vi "Read Tester.vi"(6 "Maximum Time (10000 ms)":u32=10000, 8 "error in (no error)":errorcluster, 11 "VISA resource name":refnum<visa-resource-name>) -> (0 "error out":errorcluster, 1 "Current (A)":dbl format="%^#_9g", 2 "Power (dBm)":dbl format="%^#_9g", 3 "VISA resource name out":refnum<visa-resource-name>, 5 "Frequency (Hz)":dbl format="%^#_9g")   [LabVIEW 2011, in "Agilent E5052X.lvlib"]
doc: "Reads tester mode trace data of the Frequency/Power measurement from the instrument.\n\n<b>Note: </b>\n\nThis VI only applies to when the Frequency/Power mode has been set to \"Tester Mode\" instead of \"Analyzer Mode\" through the \"Configure Measurement (Freq-Power)\" VI."
uses:
  Agilent E5052X.lvlib
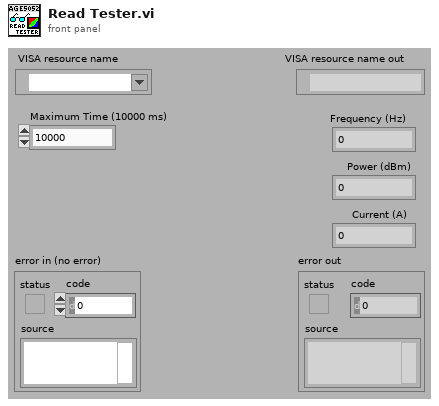
[diagram p1: front panel]
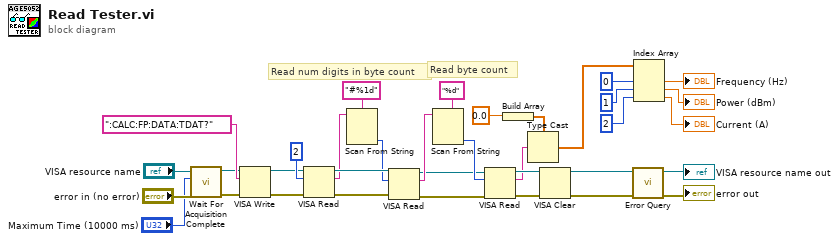
[diagram p0: block diagram]
diagram:
  # "Read num digits in byte count"
  # "Read byte count"
  n1 = call "Wait For Acquisition Complete.vi"("error in (no error)"="error in (no error)", "Maximum Time (10000)"="Maximum Time (10000 ms)", "VISA resource name"="VISA resource name") -> ("error out"=w10:errorcluster, "VISA resource name out"=w11:refnum<visa-resource-name>)  [unwired: 7 in]
  n2 = VISA Write(VISA resource name=w11, write buffer=":CALC:FP:DATA:TDAT?", error in (no error)=w10) -> (VISA resource name out=w24:refnum<visa-resource-name>, error out=w23:errorcluster)  [unwired: 1 out]
  n3 = VISA Read(VISA resource name=w24, byte count=u32 2, error in (no error)=w23) -> (VISA resource name out=w29:refnum<visa-resource-name>, read buffer=w25:string, error out=w30:errorcluster)  [unwired: 1 out]
  n4 = Scan From String(format string="#%1d", input string=w25) -> (output 1=w28:i32)  [unwired: 3 in, 3 out]
  n5 = VISA Read(VISA resource name=w29, byte count=w28, error in (no error)=w30) -> (VISA resource name out=w21:refnum<visa-resource-name>, read buffer=w27:string, error out=w20:errorcluster)  [unwired: 1 out]
  n6 = Scan From String(format string="%d", input string=w27) -> (output 1=w22:i32)  [unwired: 3 in, 3 out]
  n7 = VISA Read(VISA resource name=w21, byte count=w22, error in (no error)=w20) -> (VISA resource name out=w12:refnum<visa-resource-name>, read buffer=w2:string, error out=w13:errorcluster)  [unwired: 1 out]
  n8 = Build Array(sgl 0.0) -> (w3:sgl[])
  n9 = Type Cast(type=w3, x=w2) -> (*(type *) &x=w1:sgl[])
  n10 = VISA Clear(VISA resource name=w12, error in (no error)=w13) -> (VISA resource name out=w6:refnum<visa-resource-name>, error out=w5:errorcluster)
  n11 = call "Error Query.vi"("error in (no error)"=w5, "VISA resource name"=w6) -> ("error out"=→"error out":errorcluster, "VISA resource name out"=→"VISA resource name out":refnum<visa-resource-name>)  [unwired: 6 in, 2 out]
  n12 = Index Array(array=w1, index #1=0 ("index"), index #2=1 ("index"), index #3=2 ("index")) -> (element #1=→"Frequency (Hz)":sgl, element #2=→"Power (dBm)":sgl, element #3=→"Current (A)":sgl)
